vi "Read Touchstone File.vi"(8 "Error In":errorcluster, 11 "File Path Control":path) -> (0 "Error Out":errorcluster, 3 "Sparameters":T1[](array[typedef]))   [LabVIEW 2020]
uses:
  Instruments/Vector Network Analyzer/Controls/Sparameter cluster.ctl
  Instruments/Vector Network Analyzer/Vector Network Analyzer.lvclass
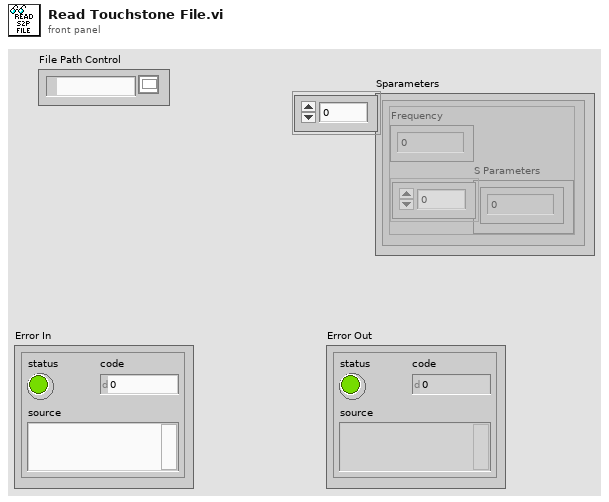
[diagram p1: front panel]
types:
  T1 = typedef "Vector Network Analyzer.lvclass/Sparameter cluster.ctl" = cluster{"Frequency":dbl, "S Parameters":cdb[]}
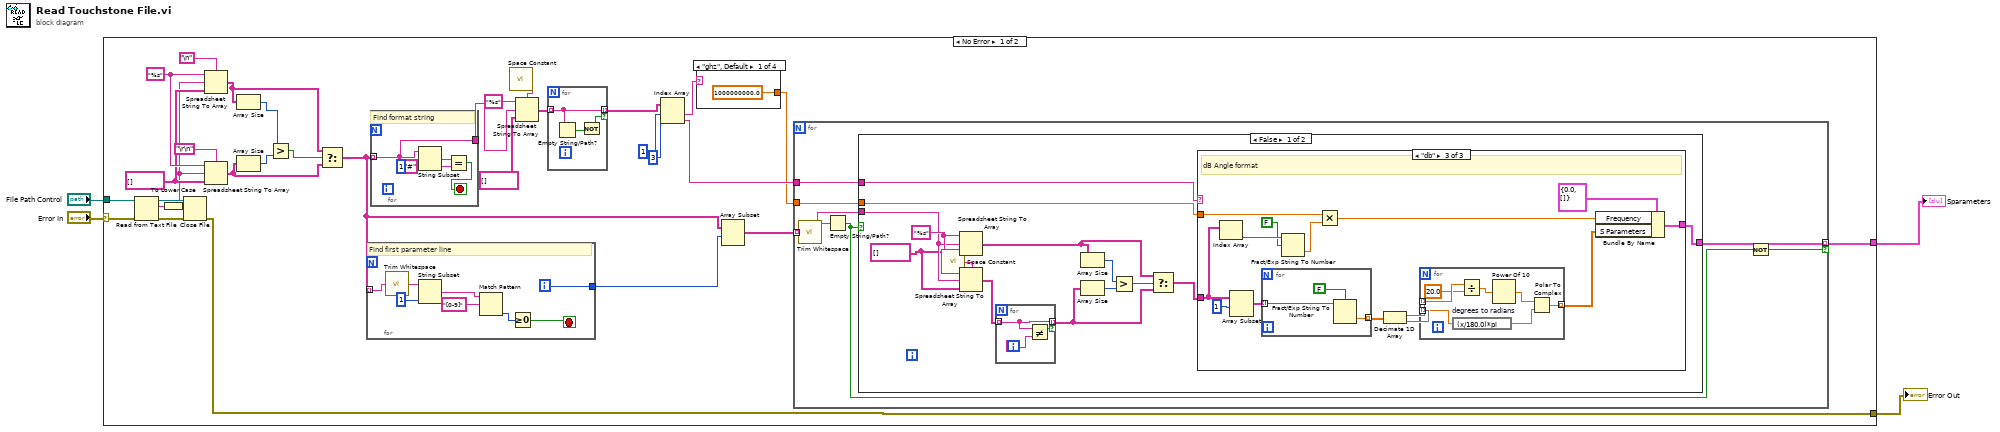
[diagram p0: block diagram]
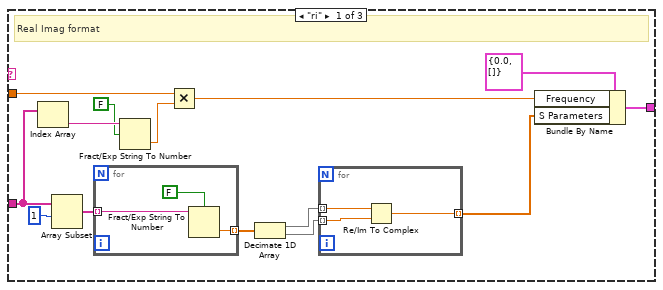
[diagram p2: hidden frame]
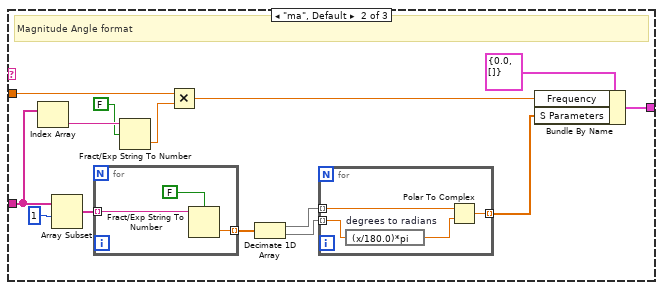
[diagram p3: hidden frame]
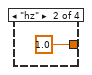
[diagram p5: hidden frame]
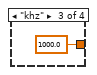
[diagram p6: hidden frame]
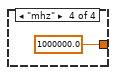
[diagram p7: hidden frame]
diagram:
  n1 = case shown="No Error" "Error In" {
    selector: "Error In" -> [w35 w145]
    tunnel: "File Path Control" -> [w34 _]
    tunnel: [w9 _] -> w2
    tunnel: [w7 w145] -> w1
    frame No Error {
      w28 = string[] []
      w30 = "%s" ("format string")
      n2 = Read from Text File(file (use dialog)=w34, error in=w35) -> (refnum out=w33:refnum<file>, text=w29:string, error out=w32:errorcluster)  [unwired: 2 in, 1 out]
      n3 = To Lower Case(string=w29) -> (all lower case string=w14:string)
      n4 = Close File(refnum=w33, error in=w32) -> (error out=w7:errorcluster)  [unwired: 1 out]
      n5 = Spreadsheet String To Array(delimiter (Tab)="\n", format string=w30, spreadsheet string=w14, array type (2D Dbl)=w28) -> (array=w23:string[])
      n6 = Spreadsheet String To Array(delimiter (Tab)="\r\n", format string=w30, spreadsheet string=w14, array type (2D Dbl)=w28) -> (array=w22:string[])
      n7 = Array Size(array=w23) -> (size(s)=w26:i32)
      n8 = Array Size(array=w22) -> (size(s)=w25:i32)
      n9 = Greater?(x=w26, y=w25) -> (0:w24:bool)
      n10 = Select(t=w23, s=w24, f=w22) -> (s? t:f=w13:string[])
      n11 = for {
        tunnel: w13 -> [w129] mode=indexing
        tunnel: [w130] -> w12
        i -> [w130]
        stop <- w131 stop-if-true
        # "Find first parameter line"
        n12 = call <vilib>:"Trim Whitespace.vi"("string"=w129) -> ("trimmed string"=w128:string)  [unwired: 1 in]
        n13 = String Subset(string=w128, length (rest)=1 ("length (rest)")) -> (substring=w133:string)  [unwired: 1 in]
        n14 = Match Pattern(string=w133, regular expression="[0-9]") -> (offset past match=w132:i32)  [unwired: 1 in, 3 out]
        n15 = Greater Or Equal To 0?(x=w132) -> (x >= 0?=w131:bool)
      }
      n16 = for {
        tunnel: w13 -> [w140] mode=indexing
        tunnel: [w140] -> w20
        stop <- w141 stop-if-true
        # "Find format string"
        n17 = String Subset(string=w140, length (rest)=1 ("length (rest)")) -> (substring=w143:string)  [unwired: 1 in]
        n18 = Equal?(x=w143, y="#") -> (x = y?=w141:bool)
      }
      n19 = call <vilib>:"Space Constant.vi"() -> ("String"=w18:string)
      n20 = Spreadsheet String To Array(delimiter (Tab)=w18, format string="%s", spreadsheet string=w20, array type (2D Dbl)=string[] []) -> (array=w5:string[])
      n21 = for {
        tunnel: [w38] -> w6 mode=indexing if=w36
        tunnel: w5 -> [w38] mode=indexing
        n22 = Empty String/Path?(string/path=w38) -> (empty?=w37:bool)
        n23 = Not(x=w37) -> (.not. x?=w36:bool)
      }
      n24 = Index Array(array=w6, index #1=1 ("index"), index #2=3 ("index")) -> (element #1=w15:string, element #2=w10:string)
      n25 = case shown="\"ghz\", Default" w15 {
        tunnel: [1000000000.0 1.0 1000.0 1000000.0] -> w8
        frame "ghz", Default {
        }
        frame "hz" {
        }
        frame "khz" {
        }
        frame "mhz" {
        }
      }
      n26 = Array Subset(array=w13, index=w12) -> (w11:string[])  [unwired: 1 in]
      n27 = for {
        tunnel: w11 -> [w44] mode=indexing
        tunnel: w10 -> [w45]
        tunnel: [w43] -> w9 mode=indexing if=w40
        tunnel: w8 -> [w42]
        n28 = call <vilib>:"Trim Whitespace.vi"("string"=w44) -> ("trimmed string"=w39:string)  [unwired: 1 in]
        n29 = Empty String/Path?(string/path=w39) -> (empty?=w41:bool)
        n30 = case shown="False" w41 {
          tunnel: w45 -> [w59 _]
          tunnel: w39 -> [w54 _]
          tunnel: [w58 _] -> w43
          tunnel: w42 -> [w57 _]
          frame False {
            w55 = "%s" ("format string")
            w53 = string[] []
            n31 = call <vilib>:"Space Constant.vi"() -> ("String"=w56:string)
            n32 = Spreadsheet String To Array(format string=w55, spreadsheet string=w54, array type (2D Dbl)=w53) -> (array=w49:string[])  [unwired: 1 in]
            n33 = Spreadsheet String To Array(delimiter (Tab)=w56, format string=w55, spreadsheet string=w54, array type (2D Dbl)=w53) -> (array=w47:string[])
            n34 = for {
              tunnel: w47 -> [w61] mode=indexing
              tunnel: [w61] -> w46 mode=indexing if=w60
              n35 = Not Equal?(x=w61, y="") -> (x != y?=w60:bool)
            }
            n36 = Array Size(array=w49) -> (size(s)=w51:i32)
            n37 = Array Size(array=w46) -> (size(s)=w52:i32)
            n38 = Greater?(x=w51, y=w52) -> (0:w50:bool)
            n39 = Select(t=w49, s=w50, f=w46) -> (s? t:f=w48:string[])
            n40 = case shown="\"db\"" w59 {
              tunnel: w48 -> [w73 w93 w114]
              tunnel: [w65 w85 w106] -> w58
              tunnel: w57 -> [w63 w83 w104]
              frame "ri" {
                # "Real Imag format"
                n41 = Index Array(array=w73) -> (element=w76:string)  [unwired: 1 in]
                n42 = Array Subset(array=w73, index=1) -> (w71:string[])  [unwired: 1 in]
                n43 = for {
                  tunnel: w71 -> [w82] mode=indexing
                  tunnel: [w80] -> w70 mode=indexing
                  n44 = Fract/Exp String To Number(use system decimal point (T)=FALSE, string=w82) -> (number=w80:dbl)  [unwired: 2 in, 1 out]
                }
                n45 = Fract/Exp String To Number(use system decimal point (T)=FALSE, string=w76) -> (number=w74:dbl)  [unwired: 2 in, 1 out]
                n46 = Multiply(x=w63, y=w74) -> (x*y=w64:dbl)
                n47 = Decimate 1D Array(w70) -> (w69:dbl[], w68:dbl[])
                n48 = for {
                  tunnel: w69 -> [w79] mode=indexing
                  tunnel: w68 -> [w78] mode=indexing
                  tunnel: [w77] -> w67 mode=indexing
                  n49 = Re/Im To Complex(1:w78, 2:w79) -> (0:w77:cdb)
                }
                n50 = Bundle By Name(cluster=T1 {"Frequency"=0.0, "S Parameters"=[]} ("S Parameters"), "Frequency"=w64, "S Parameters"=w67) -> (w65:T1)
              }
              frame "ma", Default {
                # "Magnitude Angle format"
                n51 = Index Array(array=w93) -> (element=w96:string)  [unwired: 1 in]
                n52 = Array Subset(array=w93, index=1) -> (w91:string[])  [unwired: 1 in]
                n53 = for {
                  tunnel: w91 -> [w103] mode=indexing
                  tunnel: [w101] -> w90 mode=indexing
                  n54 = Fract/Exp String To Number(use system decimal point (T)=FALSE, string=w103) -> (number=w101:dbl)  [unwired: 2 in, 1 out]
                }
                n55 = Fract/Exp String To Number(use system decimal point (T)=FALSE, string=w96) -> (number=w94:dbl)  [unwired: 2 in, 1 out]
                n56 = Multiply(x=w83, y=w94) -> (x*y=w84:dbl)
                n57 = Decimate 1D Array(w90) -> (w89:dbl[], w88:dbl[])
                n58 = for {
                  tunnel: w89 -> [w100] mode=indexing
                  tunnel: w88 -> [w99] mode=indexing
                  tunnel: [w98] -> w87 mode=indexing
                  n59 = expression code="(x/180.0)*pi" "degrees to radians"(w99) -> (w97:dbl)
                  n60 = Polar To Complex(1:w97, 2:w100) -> (0:w98:cdb)
                }
                n61 = Bundle By Name(cluster=T1 {"Frequency"=0.0, "S Parameters"=[]} ("S Parameters"), "Frequency"=w84, "S Parameters"=w87) -> (w85:T1)
              }
              frame "db" {
                # "dB Angle format"
                n62 = Index Array(array=w114) -> (element=w117:string)  [unwired: 1 in]
                n63 = Array Subset(array=w114, index=1) -> (w112:string[])  [unwired: 1 in]
                n64 = for {
                  tunnel: w112 -> [w127] mode=indexing
                  tunnel: [w125] -> w111 mode=indexing
                  n65 = Fract/Exp String To Number(use system decimal point (T)=FALSE, string=w127) -> (number=w125:dbl)  [unwired: 2 in, 1 out]
                }
                n66 = Fract/Exp String To Number(use system decimal point (T)=FALSE, string=w117) -> (number=w115:dbl)  [unwired: 2 in, 1 out]
                n67 = Multiply(x=w104, y=w115) -> (x*y=w105:dbl)
                n68 = Decimate 1D Array(w111) -> (w110:dbl[], w109:dbl[])
                n69 = for {
                  tunnel: w110 -> [w124] mode=indexing
                  tunnel: w109 -> [w123] mode=indexing
                  tunnel: [w122] -> w108 mode=indexing
                  n70 = expression code="(x/180.0)*pi" "degrees to radians"(w123) -> (w121:dbl)
                  n71 = Divide(x=w124, y=20.0) -> (x/y=w119:dbl)
                  n72 = Power Of 10(x=w119) -> (10^x=w118:dbl)
                  n73 = Polar To Complex(1:w121, 2:w118) -> (0:w122:cdb)
                }
                n74 = Bundle By Name(cluster=T1 {"Frequency"=0.0, "S Parameters"=[]} ("S Parameters"), "Frequency"=w105, "S Parameters"=w108) -> (w106:T1)
              }
            }
          }
          frame True {
          }
        }
        n75 = Not(x=w41) -> (.not. x?=w40:bool)
      }
    }
    frame Error {
    }
  }
  "Error Out" <- w1
  "Sparameters" <- w2
